vi "Cal File Read Data Section.vi"(7 "Band Selection":i32=-1, 8 "error in (no error)":errorcluster, 10 "DATA SECTION":T1, 11 "CAL File Path":path) -> (0 "error out":errorcluster, 3 "DATA":dbl[][](array[numeric]))   [LabVIEW 2011]
uses:
  Module Cal File Section.ctl
  <vilib>/Utility/config.llb/NI_LVConfig.lvlib
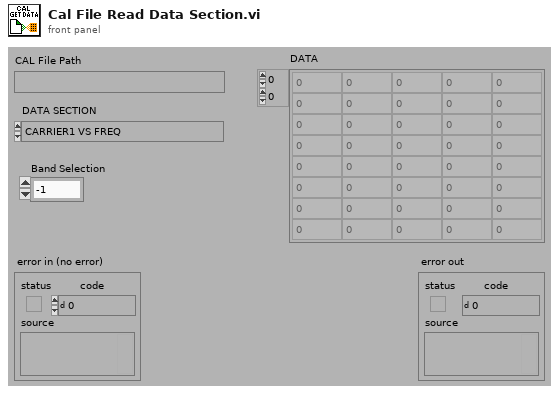
[diagram p1: front panel]
types:
  T1 = typedef "Module Cal File Section.ctl" = enum16{"CARRIER1 VS FREQ", "CARRIER2 VS FREQ", "PAD1 VS FREQUENCY", "PAD2 VS FREQUENCY", "RX POWER VS FREQUENCY", "PORT 3 VS ATTENUATION", "PORT 3 VS FREQUENCY", "HIGH POWER PAD VS FREQUENCY", "D1 VS ATTENUATION", "D1 VS FREQUENCY", "D2 VS ATTENUATION", "D2 VS FREQUENCY", "D1 LOSS VS FREQUENCY", "D2 LOSS VS FREQUENCY", "RX REVERSE", "RX FORWARD", "RX AUXILIARY", "TXA", "TXB", "TXC", "RXA", "RXB", "RXC", "RXD", "RXE", "RXF"}
  T2 = typedef "NI_LVConfig.lvlib/Config Data RefNum.ctl" = refnum<k1>
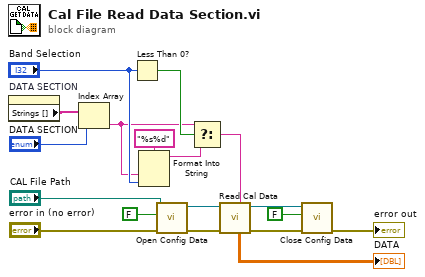
[diagram p0: block diagram]
diagram:
  n1 = property on="DATA SECTION" class="Enum (strict)"() -> ("Strings []"=w17:string[])  [unwired: 2 in, 2 out]
  n2 = Index Array(array=w17, index="DATA SECTION") -> (element=w3:string)
  n3 = Less Than 0?(x="Band Selection") -> (x < 0?=w4:bool)
  n4 = Format Into String(format string="%s%d", w3, "Band Selection") -> (resulting string=w2:string)  [unwired: 2 in, 1 out]
  n5 = call <vilib>:"Open Config Data.vi"("error in (no error)"="error in (no error)", "create file if necessary (T)"=FALSE ("create file if necessary? (T)"), "configuration file path"="CAL File Path") -> ("error out"=w15:errorcluster, "refnum"=w13:T2)  [unwired: 6 in, 1 out]
  n6 = Select(t=w3, s=w4, f=w2) -> (s? t:f=w1:string)
  n7 = call "Read Cal Data.vi"("Cal Ref"=w13, "error in (no error)"=w15, "SECTION (\"\")"=w1) -> ("DATA"=→"DATA":dbl[][], "dup Cal Ref"=w11:T2, "error out"=w12:errorcluster)  [unwired: 4 out]
  n8 = call <vilib>:"Close Config Data.vi"("error in (no error)"=w12, "write file if changed (T)"=FALSE ("write configuration file? (T)"), "refnum"=w11) -> ("error out"=→"error out":errorcluster)  [unwired: 8 out]
